vi "Task_code_SYNCH.vi"(6 "SoundWave":waveform(dbl), 7 "CardioSynchExperimentalMatrix":i32[][](array[numeric]), 8 "StimIndice":i16, 9 "Bloc":i8, 10 "TriggerPort":refnum<visa-resource-name>, 11 "Rpeak_detected":bool) -> (1 "StimIndice_Next":i16, 2 "TriggerPort":refnum<visa-resource-name>)   [LabVIEW 2022 SP3]
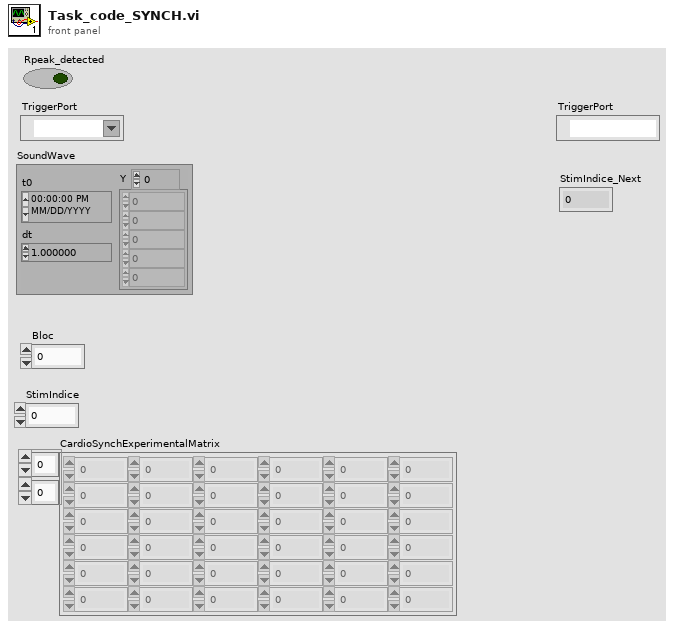
[diagram p1: front panel]
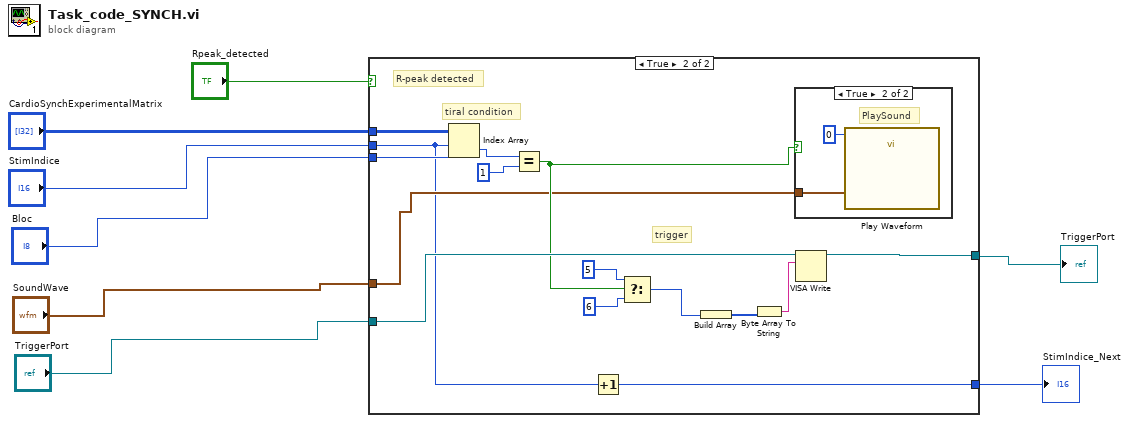
[diagram p0: block diagram]
diagram:
  n1 = case shown="True" "Rpeak_detected" {
    tunnel: "CardioSynchExperimentalMatrix" -> [_ w25]
    tunnel: "StimIndice" -> [w9 w12]
    tunnel: "Bloc" -> [_ w24]
    tunnel: "TriggerPort" -> [w10 w17]
    tunnel: [w10 w16] -> w7
    tunnel: "SoundWave" -> [_ w13]
    tunnel: [w9 w11] -> w1
    frame False {
      # "no R-peak"
    }
    frame True {
      # "trigger"
      # "tiral condition"
      # "R-peak detected"
      n2 = Index Array(array=w25, index (row)=w12, index (col)=w24) -> (element=w23:i32)
      n3 = Equal?(x=w23, y=1) -> (x = y?=w14:bool)
      n4 = Increment(x=w12) -> (x+1=w11:i16)
      n5 = Select(t=i8 5, s=w14, f=i8 6 ("t")) -> (s? t:f=w15:i8)
      n6 = Build Array(w15) -> (w19:i8[])
      n7 = Byte Array To String(unsigned byte array=w19) -> (string=w18:string)
      n8 = case shown="True" w14 {
        tunnel: w13 -> [_ w27]
        frame False {
        }
        frame True {
          # "PlaySound"
          n9 = call "Play Waveform"("Device"=u32 0, "Data"=w27) -> ()  [unwired: 17 in, 1 out]
        }
      }
      n10 = VISA Write(VISA resource name=w17, write buffer=w18) -> (VISA resource name out=w16:refnum<visa-resource-name>)  [unwired: 1 in, 2 out]
    }
  }
  "TriggerPort" <- w7
  "StimIndice_Next" <- w1
